vi "AutoBoxReadyWait.vi"(8 "error in (no error)":errorcluster, 11 "TimeOut (s)":dbl=99.0) -> (0 "error out":errorcluster)   [LabVIEW 2023]
doc: "Wrapper class for auto do nothing and wait\nInput:\n -- error in -- Cluster \n -- time out -- Double -- how long to wait B4 quitting\nOutput:\n -- error out -- Cluster"
uses:
  <vilib>/Utility/semaphor.llb/Obtain Semaphore Reference.vi
  <vilib>/Rock Robotics/WPI/ThirdParty/JAS_Junk/TrajLib/Timer_Reset.vi
  <vilib>/Rock Robotics/WPI/ThirdParty/JAS_Junk/TrajLib/Trajectory_Library.lvlib
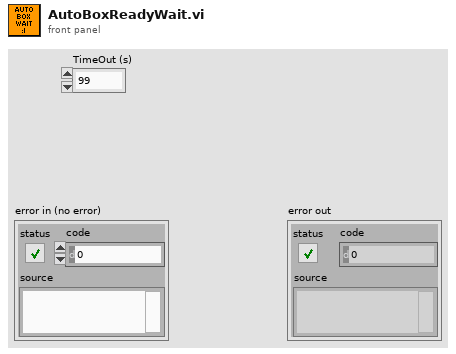
[diagram p1: front panel]
types:
  T1 = typedef "Trajectory_Library.lvlib/TIMER.ctl" = cluster{"StartTime":dbl, "Accumulated TIme":dbl, "Running":bool, "semaphore":T2}
  T2 = typedef "Semaphore RefNum" = refnum<k1>
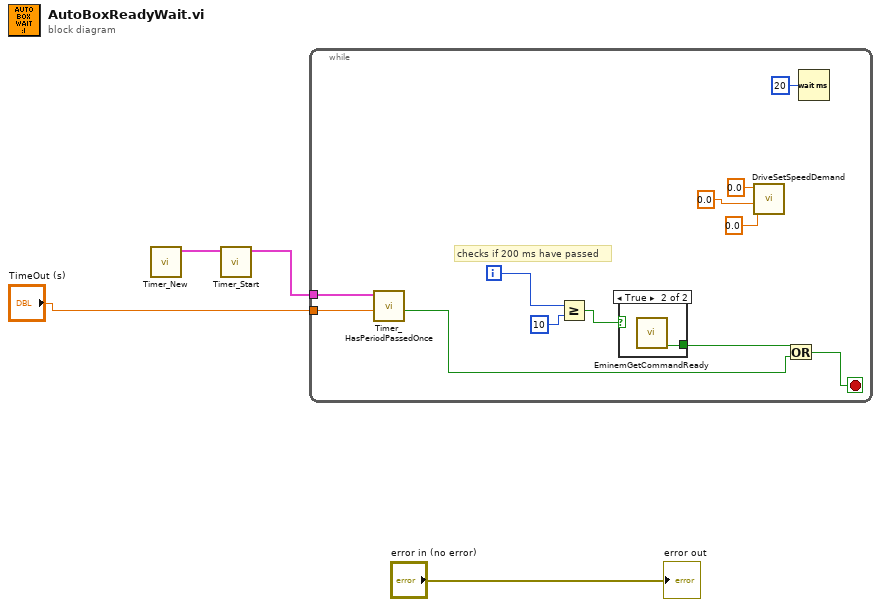
[diagram p0: block diagram]
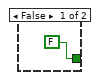
[diagram p2: hidden frame]
diagram:
  n1 = call <vilib>:"Timer_New.vi"() -> ("TIMER"=w3:T1)  [unwired: 11 in]
  n2 = call <vilib>:"Timer_Start.vi"("in Timer"=w3) -> ("out Timer"=w2:T1)  [unwired: 10 in]
  n3 = while {
    tunnel: w2 -> [w16]
    tunnel: "TimeOut (s)" -> [w15]
    i -> [w7]
    stop <- w8 stop-if-true
    # "checks if 200 ms have passed"
    n4 = call <vilib>:"Timer_HasPeriodPassedOnce.vi"("Period"=w15, "in Timer"=w16) -> ("Expired"=w9:bool)  [unwired: 7 in, 2 out]
    n5 = Greater Or Equal?(x=w7, y=10) -> (x >= y?=w6:bool)
    n6 = case shown="True" w6 {
      tunnel: [FALSE w18] -> w10
      frame False {
      }
      frame True {
        n7 = call "EminemGetCommandReady.vi"() -> ("BoxCommandReady"=w18:bool)  [unwired: 11 in]
      }
    }
    n8 = call "DriveSetSpeedDemand.vi"("ASpeedDemand (d/s)"=0.0 ("RSpeedDemand (ft/s)"), "YSpeedDemand (ft/s)"=0.0 ("RSpeedDemand (ft/s)"), "XSpeedDemand (ft/s)"=0.0 ("LSpeedDemand (ft/s)")) -> ()  [unwired: 9 in]
    n9 = Or(x=w10, y=w9) -> (x .or. y?=w8:bool)
    n10 = Wait (ms)(milliseconds to wait=u32 20) -> ()  [unwired: 1 out]
  }
  "error out" <- "error in (no error)"
